vi "PotentialADP.vi"() -> ()   [LabVIEW 2019]
uses:
  <vilib>/Instr/_visa.llb/VISA Configure Serial Port (Instr).vi
  <vilib>/Utility/file.llb/Write Delimited Spreadsheet (string).vi
  <vilib>/Utility/file.llb/Write Delimited Spreadsheet (DBL).vi
  <vilib>/ptbypt/NI_PtbyPt.lvlib
panel:
  in  "Arduino Power":bool
  in  "C":dbl
  in  "A":dbl=0.0073
  in  "B":dbl=-2.0616
  out "Water Offset":dbl
  out "UV Offset":dbl
  out "Lux Offset":dbl
  out "HumidOffset":dbl
  in  "Calibration Mode":bool
  out "Present (s)":dbl
  out "Elapsed Time (s)":dbl
  out "Water Warning":bool
  out "Water Alarm":bool
  out "Water Level":dbl
  out "UV Warning":bool
  out "UV Alarm":bool
  out "UV Value":dbl
  out "Lux Chart":dbl(graph)
  out "Lux Alarm":bool
  out "Lux Warning":bool
  out "Lux Value":dbl
  out "Data: Time, Humidity, Temperature, UV, Lux, Water Level":dbl[][](array[numeric])
  in  "Temp Bias":dbl
  out "Temp. Mean":dbl format="%0.2f"
  out "Temp Chart":dbl(graph)
  out "Temp Alarm":bool
  out "Temp Warning":bool
  out "Temperature (F)":dbl
  out "Humidity Chart":dbl(graph)
  out "Humid Alarm":bool
  out "Humid Warning":bool
  out "Humidity":dbl
  in  "Operational Mode":bool
  in  "Arduino COM Port":refnum<visa-resource-name>="COM3"
  in  "?":bool
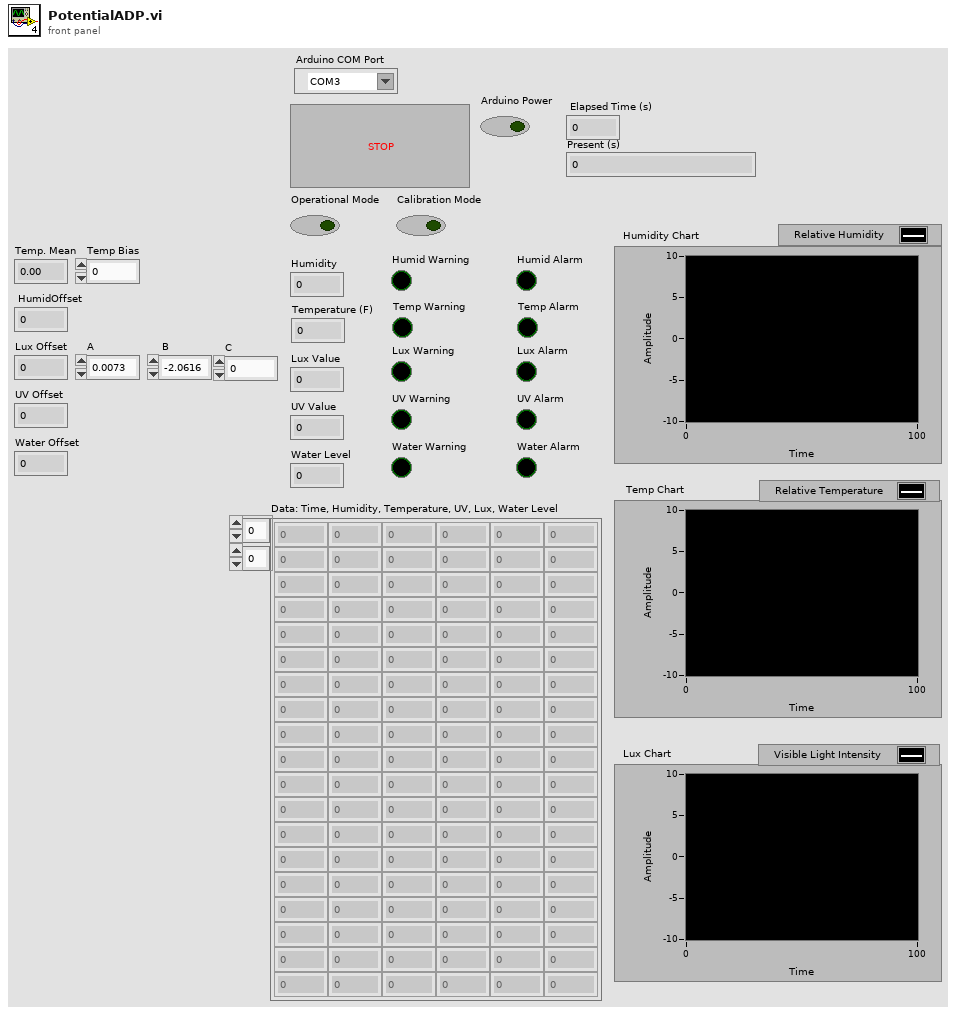
[diagram p1: front panel]
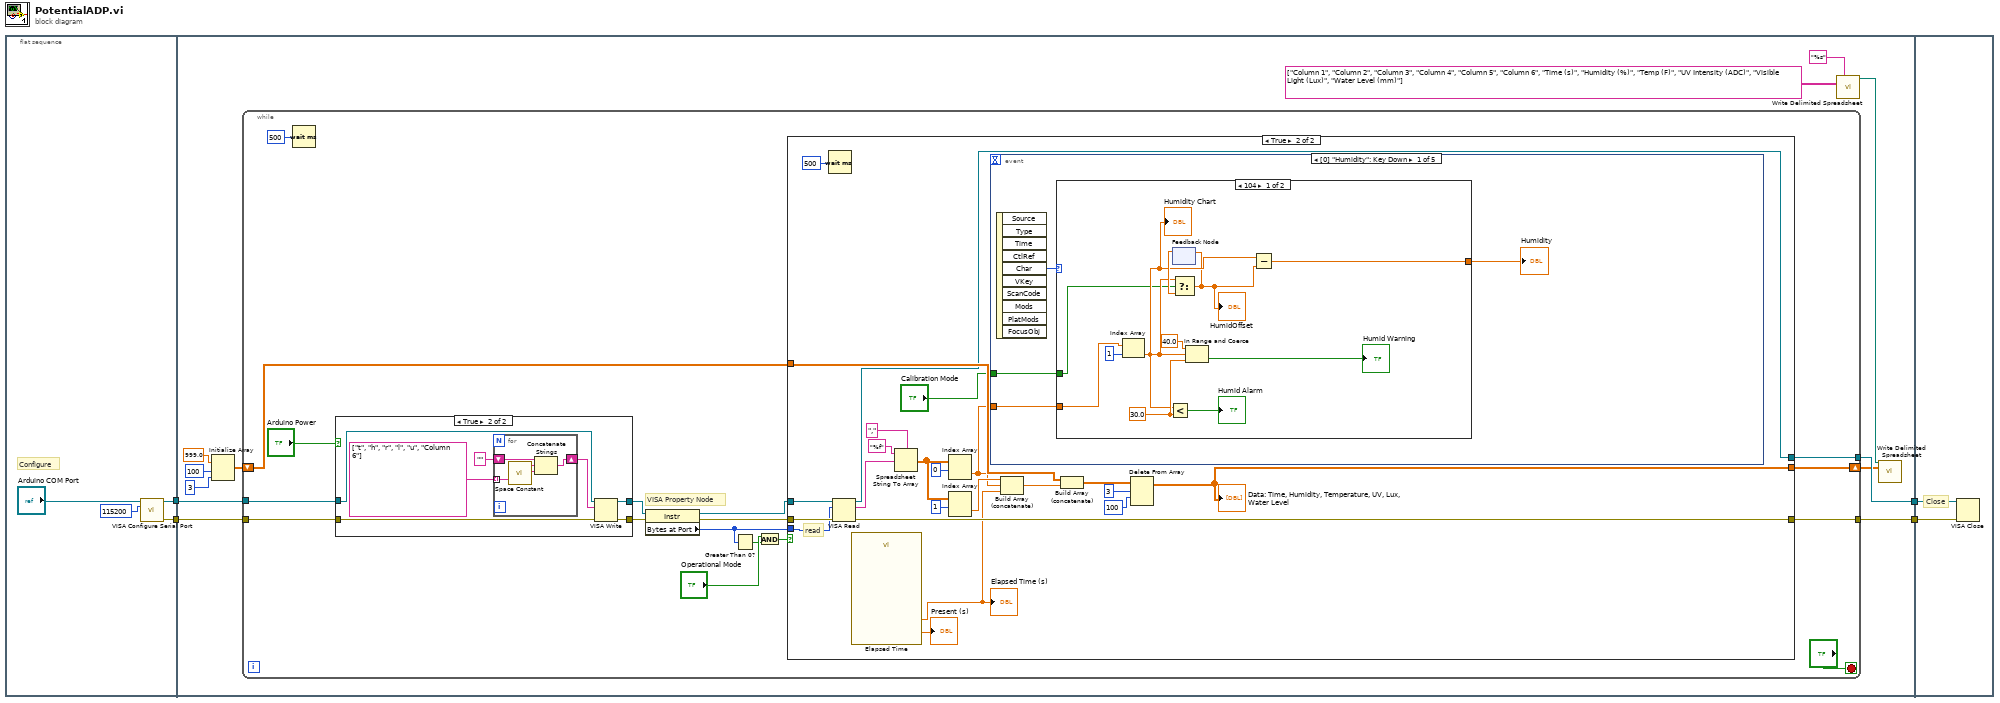
[diagram p0: block diagram]
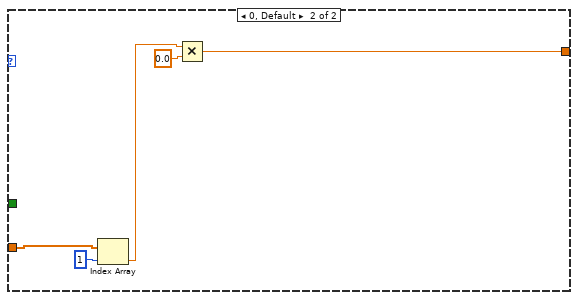
[diagram p4: hidden frame]
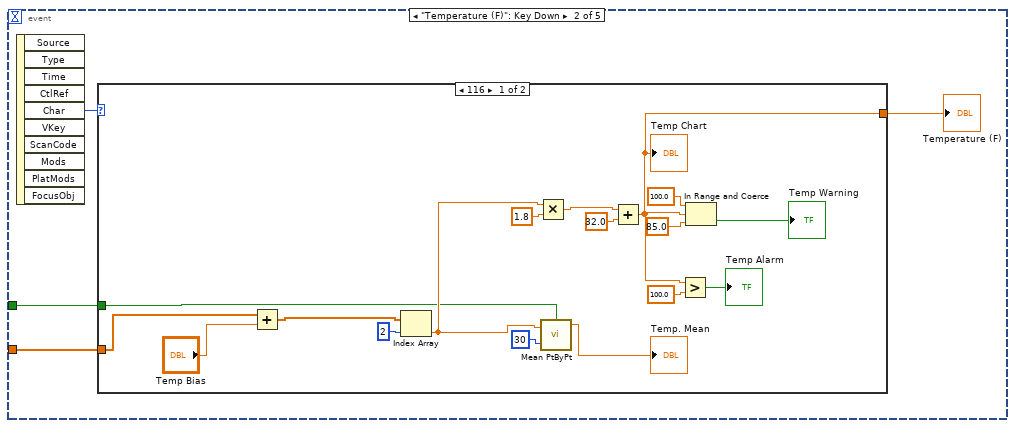
[diagram p5: hidden frame]
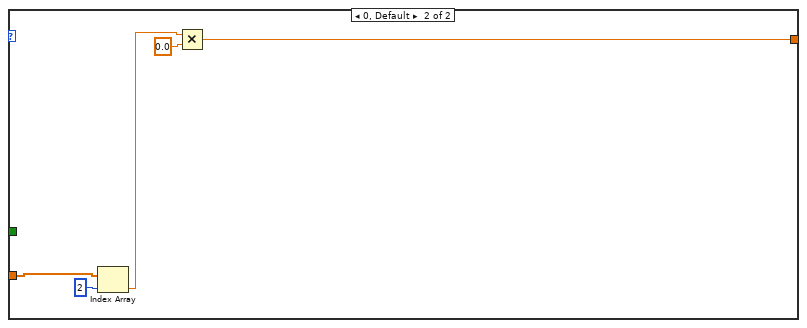
[diagram p6: hidden frame]
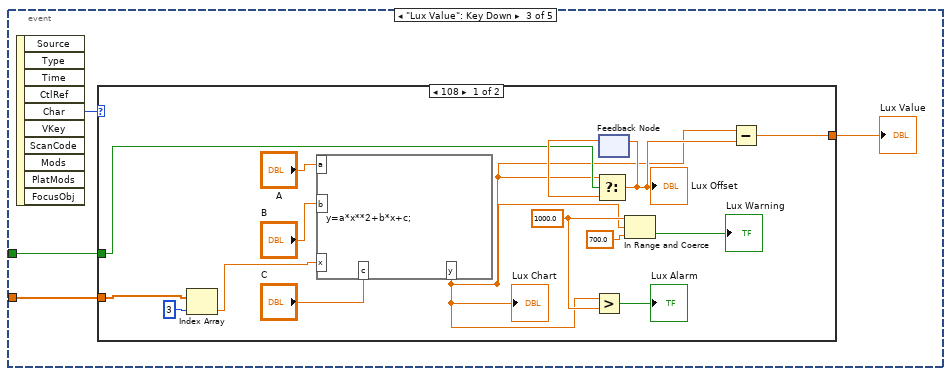
[diagram p7: hidden frame]
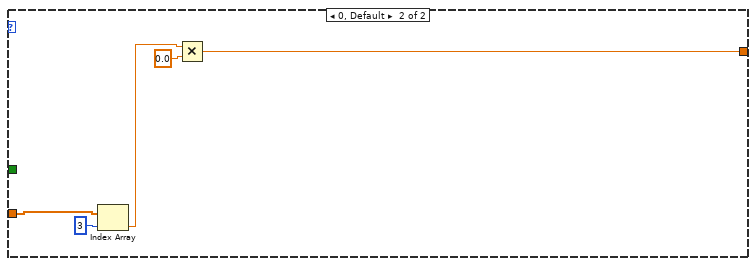
[diagram p8: hidden frame]
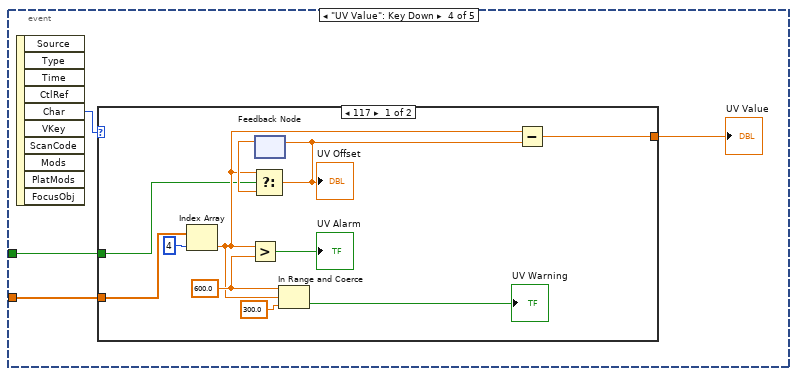
[diagram p9: hidden frame]
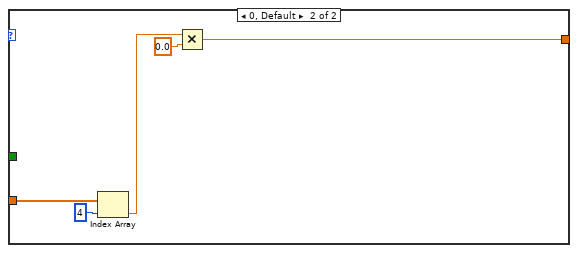
[diagram p10: hidden frame]
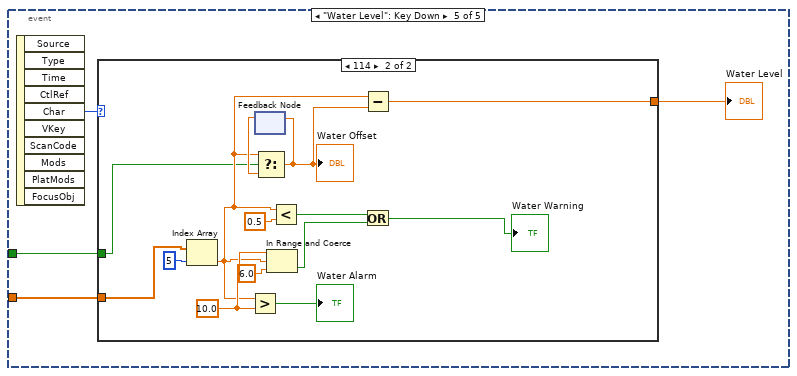
[diagram p11: hidden frame]
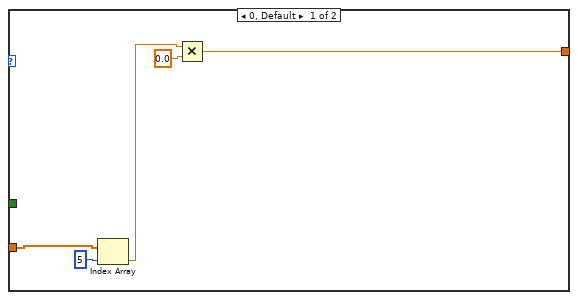
[diagram p12: hidden frame]
diagram:
  n1 = flat-sequence {
    tunnel: [w5] -> w4
    tunnel: [w6] -> w3
    tunnel: w4 -> [w20]
    tunnel: [w19] -> w2
    tunnel: w3 -> [w18]
    tunnel: [w17] -> w1
    tunnel: w2 -> [w191]
    tunnel: w1 -> [w190]
    frame #0 {
      # "Configure"
      n2 = call-poly "VISA Configure Serial Port"("VISA resource name"="Arduino COM Port", "baud rate (9600)"=u32 115200) -> ("VISA resource name out"=w5:refnum<visa-resource-name>, "error out"=w6:errorcluster)  [unwired: 12 in]
    }
    frame #1 {
      n3 = Initialize Array(999.0 ("element"), 100 ("dimension size"), 3 ("dimension size")) -> (w13:dbl[][])
      n4 = while {
        tunnel: w20 -> [w24]
        tunnel: [w28] -> w19
        tunnel: w18 -> [w25]
        tunnel: [w29] -> w17
        shift-right: [w27] -> w9
        shift-left: w13 -> [w31]
        stop <- "?" stop-if-true
        # "VISA Property Node"
        n5 = Wait (ms)(milliseconds to wait=u32 500) -> ()  [unwired: 1 out]
        n6 = case shown="True" "Arduino Power" {
          tunnel: w25 -> [w38 w46]
          tunnel: w24 -> [w39 w45]
          tunnel: [w39 w44] -> w23
          tunnel: [w38 w43] -> w22
          frame False {
          }
          frame True {
            n7 = for {
              shift-right: [w49] -> w42
              shift-left: "" -> [w47]
              tunnel: string[] ["t", "h", "r", "l", "u", "Column 6"] ("2D data") -> [w48] mode=indexing
              n8 = call <vilib>:"Space Constant.vi"() -> ("String"=w50:string)
              n9 = Concatenate Strings(w47, w48, w50) -> (w49:string)
            }
            n10 = VISA Write(VISA resource name=w45, write buffer=w42, error in (no error)=w46) -> (VISA resource name out=w44:refnum<visa-resource-name>, error out=w43:errorcluster)  [unwired: 1 out]
          }
        }
        n11 = property class="Instr"(reference=w23, error in=w22) -> (reference out=w33:refnum<visa-resource-name>, error out=w34:errorcluster, "Bytes at Port"=w32:u32)
        n12 = Greater Than 0?(x=w32) -> (x > 0?=w35:bool)
        n13 = And(x="Operational Mode", y=w35) -> (x .and. y?=w26:bool)
        n14 = case shown="True" w26 {
          tunnel: w34 -> [w52 w76]
          tunnel: w33 -> [w51 w74]
          tunnel: w32 -> [_ w75]
          tunnel: w31 -> [w53 w65]
          tunnel: [w52 w62] -> w29
          tunnel: [w51 w61] -> w28
          tunnel: [w53 w57] -> w27
          frame False {
          }
          frame True {
            # "read"
            n15 = Wait (ms)(milliseconds to wait=u32 500) -> ()  [unwired: 1 out]
            n16 = VISA Read(VISA resource name=w74, byte count=w75, error in (no error)=w76) -> (VISA resource name out=w61:refnum<visa-resource-name>, read buffer=w73:string, error out=w62:errorcluster)  [unwired: 1 out]
            n17 = call "Elapsed Time"() -> ("Present (s)"=→"Present (s)":dbl, "Elapsed Time (s)"=w56:dbl)  [unwired: 12 in, 6 out]
            "Elapsed Time (s)" <- w56
            n18 = Spreadsheet String To Array(delimiter (Tab)=",", format string="%f", spreadsheet string=w73) -> (array=w70:dbl[][])  [unwired: 1 in]
            n19 = Index Array(array=w70, index (row)=0) -> (element=w64:dbl[])  [unwired: 1 in]
            n20 = Index Array(array=w70, index (row)=1) -> (element=w67:dbl[])  [unwired: 1 in]
            n21 = event shown="[0] \"Humidity\": Key Down" {
              selector: _ -> [_ _ _ _ _]
              dyn-events: _ -> [_ _ _ _ _]
              timeout: _ -> [_ _ _ _ _]
              tunnel: w64 -> [w79 w100 w126 w150 w170]
              tunnel: "Calibration Mode" -> [w77 w97 w123 w147 w167]
              event "Humidity": Key Down {
                n22 = event-data() -> ("Char"=w80:i16)  [unwired: 1 in, 9 out]
                n23 = case shown="104" w80 {
                  tunnel: w79 -> [w86 w95]
                  tunnel: [w85 w92] -> w78
                  tunnel: w77 -> [w81 _]
                  frame 104 {
                    w88 = 30.0 ("y")
                    n24 = Index Array(array=w86, index=1) -> (element=w83:dbl)
                    "Humidity Chart" <- w83
                    n25 = Less?(x=w83, y=w88) -> (x < y?=→"Humid Alarm":bool)
                    n26 = feedback #1() -> (w84:dbl)  [unwired: 1 in]
                    n27 = Select(t=w83, s=w81, f=w84) -> (s? t:f=w82:dbl)
                    "HumidOffset" <- w82
                    n28 = feedback-in #1(w82) -> ()
                    n29 = In Range and Coerce(upper limit=40.0 ("y"), x=w83, lower limit=w88) -> (In Range?=→"Humid Warning":bool)  [unwired: 1 out]
                    n30 = Subtract(x=w83, y=w82) -> (x-y=w85:dbl)
                  }
                  frame 0, Default {
                    n31 = Index Array(array=w95, index=1) -> (element=w94:dbl)
                    n32 = Multiply(x=w94, y=0.0) -> (x*y=w92:dbl)
                  }
                }
                "Humidity" <- w78
              }
              event "Temperature (F)": Key Down {
                n33 = event-data() -> ("Char"=w99:i16)  [unwired: 1 in, 9 out]
                n34 = case shown="116" w99 {
                  tunnel: w100 -> [w104 w121]
                  tunnel: [w102 w119] -> w98
                  tunnel: w97 -> [w101 _]
                  frame 116 {
                    n35 = Add(x=w104, y="Temp Bias") -> (x+y=w103:dbl[])
                    n36 = Index Array(array=w103, index=2) -> (element=w106:dbl)
                    n37 = Multiply(x=w106, y=1.8) -> (x*y=w109:dbl)
                    n38 = call <vilib>:"Mean PtByPt.vi"("x"=w106, "sample length"=30, "initialize"=w101) -> ("mean"=→"Temp. Mean":dbl)  [unwired: 1 in, 1 out]
                    n39 = Add(x=w109, y=32.0) -> (x+y=w102:dbl)
                    "Temp Chart" <- w102
                    n40 = Greater?(x=w102, y=100.0) -> (0:→"Temp Alarm":bool)
                    n41 = In Range and Coerce(upper limit=100.0, x=w102, lower limit=85.0 ("y")) -> (In Range?=→"Temp Warning":bool)  [unwired: 1 out]
                  }
                  frame 0, Default {
                    n42 = Index Array(array=w121, index=2) -> (element=w118:dbl)
                    n43 = Multiply(x=w118, y=0.0) -> (x*y=w119:dbl)
                  }
                }
                "Temperature (F)" <- w98
              }
              event "Lux Value": Key Down {
                n44 = event-data() -> ("Char"=w125:i16)  [unwired: 1 in, 9 out]
                n45 = case shown="108" w125 {
                  tunnel: w126 -> [w136 w145]
                  tunnel: [w134 w142] -> w124
                  tunnel: w123 -> [w131 _]
                  frame 108 {
                    w139 = 1000.0 ("y")
                    n46 = Index Array(array=w136, index=3) -> (element=w137:dbl)
                    n47 = formula code="y=a*x**2+b*x+c;"("a"="A", "x"=w137, "b"="B", "c"="C") -> ("y"=w130:dbl)
                    "Lux Chart" <- w130
                    n48 = Greater?(x=w130, y=w139) -> (0:→"Lux Alarm":bool)
                    n49 = feedback #2() -> (w132:dbl)  [unwired: 1 in]
                    n50 = Select(t=w130, s=w131, f=w132) -> (s? t:f=w133:dbl)
                    "Lux Offset" <- w133
                    n51 = feedback-in #2(w133) -> ()
                    n52 = In Range and Coerce(upper limit=w139, x=w130, lower limit=700.0 ("y")) -> (In Range?=→"Lux Warning":bool)  [unwired: 1 out]
                    n53 = Subtract(x=w130, y=w133) -> (x-y=w134:dbl)
                  }
                  frame 0, Default {
                    n54 = Index Array(array=w145, index=3) -> (element=w143:dbl)
                    n55 = Multiply(x=w143, y=0.0) -> (x*y=w142:dbl)
                  }
                }
                "Lux Value" <- w124
              }
              event "UV Value": Key Down {
                n56 = event-data() -> ("Char"=w149:i16)  [unwired: 1 in, 9 out]
                n57 = case shown="117" w149 {
                  tunnel: w150 -> [w157 w162]
                  tunnel: [w155 w165] -> w148
                  tunnel: w147 -> [w151 _]
                  frame 117 {
                    w159 = 600.0 ("y")
                    n58 = Index Array(array=w157, index=4) -> (element=w152:dbl)
                    n59 = Greater?(x=w152, y=w159) -> (0:→"UV Alarm":bool)
                    n60 = feedback #3() -> (w153:dbl)  [unwired: 1 in]
                    n61 = Select(t=w152, s=w151, f=w153) -> (s? t:f=w154:dbl)
                    "UV Offset" <- w154
                    n62 = feedback-in #3(w154) -> ()
                    n63 = In Range and Coerce(upper limit=w159, x=w152, lower limit=300.0 ("y")) -> (In Range?=→"UV Warning":bool)  [unwired: 1 out]
                    n64 = Subtract(x=w152, y=w154) -> (x-y=w155:dbl)
                  }
                  frame 0, Default {
                    n65 = Index Array(array=w162, index=4) -> (element=w163:dbl)
                    n66 = Multiply(x=w163, y=0.0) -> (x*y=w165:dbl)
                  }
                }
                "UV Value" <- w148
              }
              event "Water Level": Key Down {
                n67 = event-data() -> ("Char"=w169:i16)  [unwired: 1 in, 9 out]
                n68 = case shown="114" w169 {
                  tunnel: w170 -> [w174 w181]
                  tunnel: [w171 w180] -> w168
                  tunnel: w167 -> [_ w176]
                  frame 0, Default {
                    n69 = Index Array(array=w174, index=5) -> (element=w173:dbl)
                    n70 = Multiply(x=w173, y=0.0) -> (x*y=w171:dbl)
                  }
                  frame 114 {
                    w182 = 10.0 ("y")
                    n71 = Index Array(array=w181, index=5) -> (element=w177:dbl)
                    n72 = Greater?(x=w177, y=w182) -> (0:→"Water Alarm":bool)
                    n73 = feedback #4() -> (w178:dbl)  [unwired: 1 in]
                    n74 = Select(t=w177, s=w176, f=w178) -> (s? t:f=w179:dbl)
                    "Water Offset" <- w179
                    n75 = feedback-in #4(w179) -> ()
                    n76 = In Range and Coerce(upper limit=w182, x=w177, lower limit=6.0 ("y")) -> (In Range?=w184:bool)  [unwired: 1 out]
                    n77 = Less?(x=w177, y=0.5) -> (x < y?=w187:bool)
                    n78 = Subtract(x=w177, y=w179) -> (x-y=w180:dbl)
                    n79 = Or(x=w187, y=w184) -> (x .or. y?=→"Water Warning":bool)
                  }
                }
                "Water Level" <- w168
              }
            }
            n80 = Build Array (concatenate)(w67, w64, w56) -> (w66:dbl[])
            n81 = Build Array (concatenate)(w65, w66) -> (w58:dbl[][])
            n82 = Delete From Array(array=w58, length=3, index (row)=100) -> (array with subset deleted=w57:dbl[][])  [unwired: 1 in, 1 out]
            "Data: Time, Humidity, Temperature, UV, Lux, Water Level" <- w57
          }
        }
      }
      n83 = call-poly <vilib>:"Write Delimited Spreadsheet.vi"("format (%s)"="%s", "2D data"=string[][] [["Column 1", "Column 2", "Column 3", "Column 4", "Column 5", "Column 6"], ["Time (s)", "Humidity (%)", "Temp (F)", "UV Intensity (ADC)", "Visible Light (Lux)", "Water Level (mm)"]]) -> ("new file path (Not A Path if cancelled)"=w10:path)  [unwired: 12 in, 1 out]
      n84 = call-poly <vilib>:"Write Delimited Spreadsheet.vi"("file path (dialog if empty)"=w10, "2D data"=w9) -> ()  [unwired: 12 in, 2 out]
    }
    frame #2 {
      # "Close"
      n85 = VISA Close(VISA resource name=w191, error in (no error)=w190) -> ()  [unwired: 1 out]
    }
  }
